vi "FinalizeHWI.vi"(8 "error in (no error)":errorcluster, 10 "Master Device in":refnum<class "Master Device.lvclass">, 11 "Arduino DDS in":refnum<class "Arduino DDS.lvclass">) -> (0 "error out":errorcluster, 2 "Master Device out":refnum<class "Master Device.lvclass">, 3 "Arduino DDS out":refnum<class "Arduino DDS.lvclass">)   [LabVIEW 2013, in "Arduino DDS.lvclass"]
uses:
  Arduino DDS.lvclass
  Master Device/Master Device.lvclass
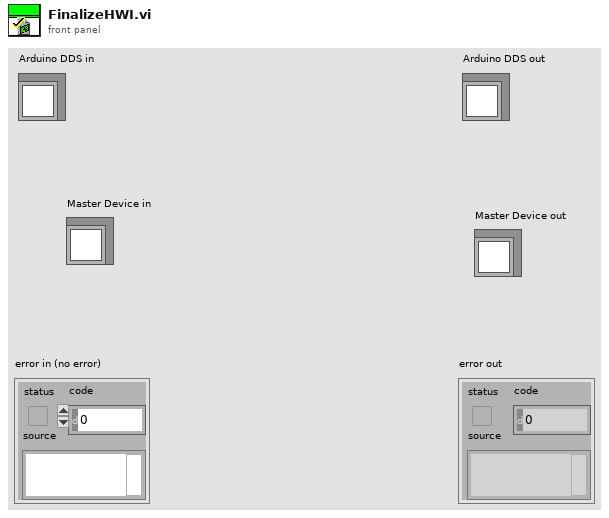
[diagram p1: front panel]
types:
  T1 = cluster{"Freq_I [MHz]":dbl[], "Phase [deg]":dbl[], "Freq_F [MHz]":dbl[], "Sweep?":bool[], "Ramp Time":dbl[], "Slaved Digital Output":bool[]}
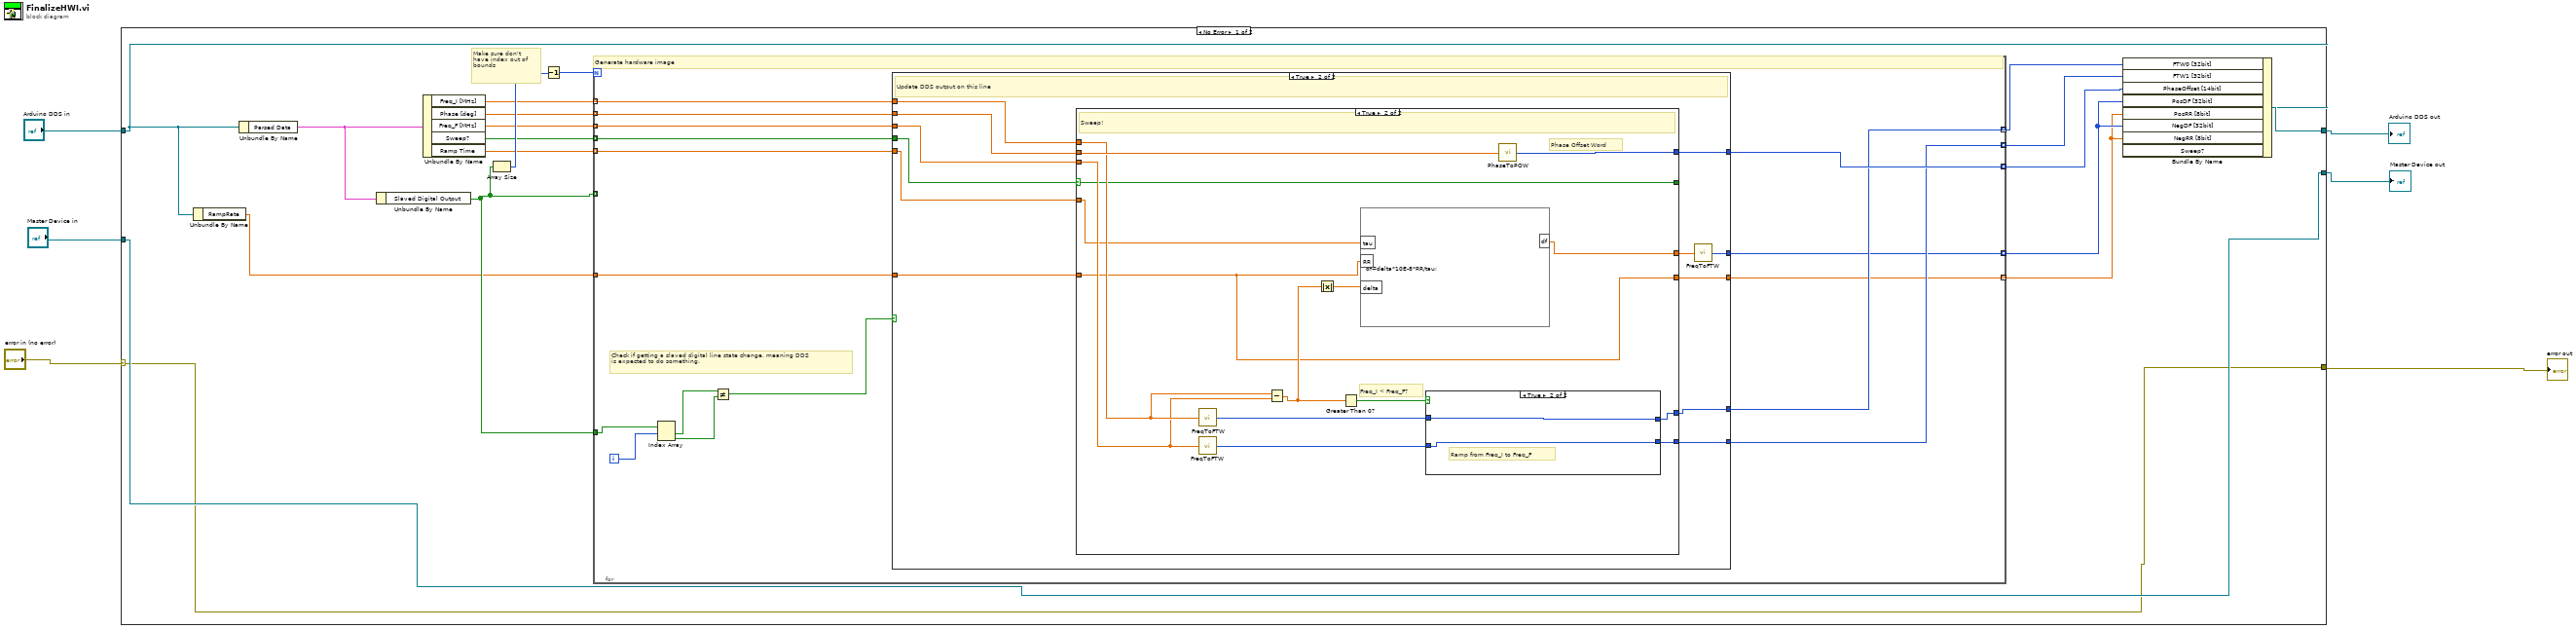
[diagram p0: block diagram]
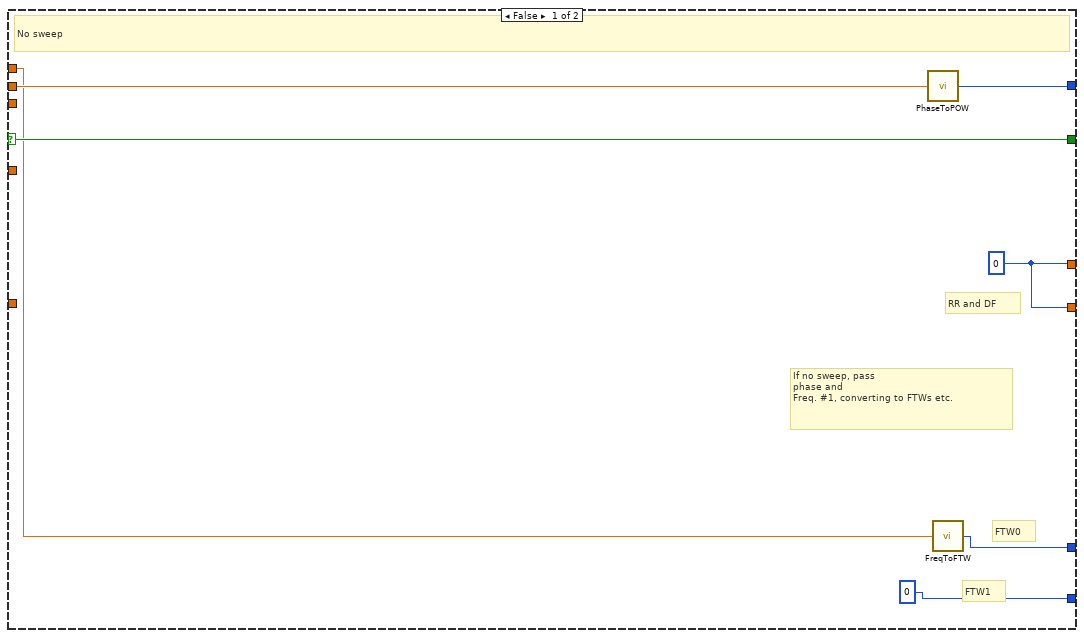
[diagram p3: hidden frame]
diagram:
  n1 = case shown="No Error" "error in (no error)" {
    selector: "error in (no error)" -> [w7 w82]
    tunnel: [w7 w82] -> w5
    tunnel: "Master Device in" -> [w8 w81]
    tunnel: [w8 w81] -> w3
    tunnel: "Arduino DDS in" -> [w15 w80]
    tunnel: [w25 w80] -> w1
    frame No Error {
      # "Make sure don't\nhave index out of\nbounds"
      n2 = Unbundle By Name(w15) -> ("RampRate"=w14:dbl)
      n3 = Unbundle By Name(w15) -> ("Parsed Data"=w22:T1)
      n4 = Unbundle By Name(w22) -> ("Slaved Digital Output"=w23:bool[])
      n5 = Unbundle By Name(w22) -> ("Freq_I [MHz]"=w21:dbl[], "Phase [deg]"=w20:dbl[], "Freq_F [MHz]"=w19:dbl[], "Sweep?"=w18:bool[], "Ramp Time"=w17:dbl[])
      n6 = Array Size(array=w23) -> (size(s)=w24:i32)
      n7 = Decrement(x=w24) -> (x-1=w16:i32)
      n8 = for {
        N: w16 -> [_]
        tunnel: w23 -> [w41]
        tunnel: w23 -> [_] mode=indexing
        tunnel: w21 -> [w36] mode=indexing
        tunnel: w20 -> [w35] mode=indexing
        tunnel: w19 -> [w34] mode=indexing
        tunnel: w18 -> [w33] mode=indexing
        tunnel: w17 -> [w32] mode=indexing
        tunnel: w14 -> [w31]
        tunnel: [w30] -> w11 mode=indexing
        tunnel: [w29] -> w13 mode=indexing
        tunnel: [w28] -> w12 mode=indexing
        tunnel: [w27] -> w10 mode=indexing
        tunnel: [w26] -> w9 mode=indexing
        i -> [w40]
        # "Check if getting a slaved digital line state change, meaning DDS\nis expected to do something."
        # "Generate hardware image"
        n9 = Index Array(array=w41, index #1=w40) -> (element #1=w39:bool, element #2=w38:bool)  [unwired: 1 in]
        n10 = Not Equal?(x=w39, y=w38) -> (x != y?=w37:bool)
        n11 = case shown="True" w37 {
          tunnel: w36 -> [_ w51]
          tunnel: w35 -> [_ w52]
          tunnel: w34 -> [_ w50]
          tunnel: w33 -> [_ w53]
          tunnel: w32 -> [_ w49]
          tunnel: w31 -> [_ w48]
          tunnel: [_ w47] -> w30
          tunnel: [_ w46] -> w29
          tunnel: [_ w45] -> w28
          tunnel: [_ w43] -> w27
          tunnel: [_ w42] -> w26
          frame False {
            # "If the line doesn't need to update DDS, don't pass through to HWI"
          }
          frame True {
            # "Update DDS output on this line"
            n12 = case shown="True" w53 {
              selector: w53 -> [w56 w63]
              tunnel: [w60 w75] -> w46
              tunnel: [0 w74] -> w45
              tunnel: [w59 w72] -> w47
              tunnel: [w58 w61] -> w42
              tunnel: [w58 w62] -> w44
              tunnel: [w56 w63] -> _
              tunnel: w52 -> [w55 w69]
              tunnel: w51 -> [w54 w68]
              tunnel: w50 -> [_ w67]
              tunnel: w49 -> [_ w64]
              tunnel: w48 -> [_ w61]
              frame False {
                w58 = 0
                # "FTW1"
                # "RR and DF"
                # "FTW0"
                # "If no sweep, pass\nphase and \nFreq. #1, converting to FTWs etc."
                # "No sweep"
                n13 = call "PhaseToPOW.vi"("Phase"=w55) -> ("POW [14bit]"=w59:u16)
                n14 = call "FreqToFTW.vi"("Frequency"=w54) -> ("FTW [32bit]"=w60:u32)
              }
              frame True {
                # "Phase Offset Word"
                # "Freq_I < Freq_F?"
                # "Sweep!"
                n15 = call "FreqToFTW.vi"("Frequency"=w67) -> ("FTW [32bit]"=w71:u32)
                n16 = call "FreqToFTW.vi"("Frequency"=w68) -> ("FTW [32bit]"=w70:u32)
                n17 = Subtract(x=w68, y=w67) -> (x-y=w66:dbl)
                n18 = Absolute Value(x=w66) -> (abs(x)=w65:dbl)
                n19 = Greater Than 0?(x=w66) -> (x > 0?=w73:bool)
                n20 = formula code="df=delta*10E-8*RR/tau;"("delta"=w65, "tau"=w64, "RR"=w61) -> ("df"=w62:dbl)
                n21 = case shown="True" w73 {
                  tunnel: [w77 w79] -> w75
                  tunnel: w70 -> [w76 w79]
                  tunnel: [w76 w78] -> w74
                  tunnel: w71 -> [w77 w78]
                  frame False {
                    # "Ramp from Freq_F to Freq_I"
                    # "Decide ramp direction"
                  }
                  frame True {
                    # "Ramp from Freq_I to Freq_F"
                  }
                }
                n22 = call "PhaseToPOW.vi"("Phase"=w69) -> ("POW [14bit]"=w72:u16)
              }
            }
            n23 = call "FreqToFTW.vi"("Frequency"=w44) -> ("FTW [32bit]"=w43:u32)
          }
        }
      }
      n24 = Bundle By Name(cluster=w15, "FTW0 [32bit]"=w13, "FTW1 [32bit]"=w12, "PhaseOffset [14bit]"=w11, "PosDF [32bit]"=w10, "PosRR [8bit]"=w9, "NegDF [32bit]"=w10, "NegRR [8bit]"=w9) -> (w25:refnum<class "Arduino DDS.lvclass">)  [unwired: 1 in]
    }
    frame Error {
    }
  }
  "error out" <- w5
  "Arduino DDS out" <- w1
  "Master Device out" <- w3
